vi "h.NET.GetNetworkIpMode.vi"(0 "Connection ID":refnum<k5>, 1 "error in":errorcluster) -> (2 "Connection ID":refnum<k5>, 3 "Network Mode":T1, 4 "Message":string, 5 "error out":errorcluster)   [LabVIEW 2016, in "h.Library.lvlib"]
doc: "This vi retrieves the current network settings.\n\n<b>Connection ID</b> - is a network connection refnum that uniquely identifies the TCP connection\n<b>error in</b> - describes error conditions that occur before this node runs. This input provides standard error functionality\n<b>Connection ID out</b> - returns the same value as connection ID\n<b>Network Mode</b> - returned network mode (either Static or DHCP)\n<b>Message</b> - human readable messages returned by the executed command\n<b>error out</b> - contains error information. This output provides standard error out functionality."
uses:
  h.Library.lvlib
  CTL/h.NET.NetworkMode.ctl
panel:
  # "Hyperion Get Network Configuration Mode"
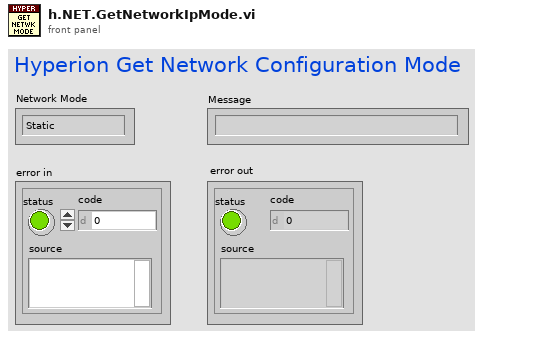
[diagram p1: front panel]
types:
  T1 = typedef "h.Library.lvlib/h.NET.NetworkMode.ctl" = enum8{"Static", "DHCP"}
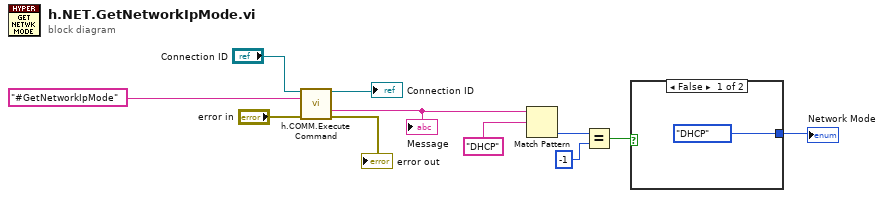
[diagram p0: block diagram]
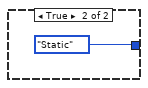
[diagram p2: hidden frame]
diagram:
  n1 = call "h.COMM.Execute Command.vi"("Connection ID"="Connection ID", "Command"="#GetNetworkIpMode", "error in"="error in") -> ("Connection ID out"=→"Connection ID":refnum<k5>, "Message"=w6:string, "error out"=→"error out":errorcluster)  [unwired: 5 in, 5 out]
  "Message" <- w6
  n2 = Match Pattern(string=w6, regular expression="DHCP" ("search string")) -> (offset past match=w4:i32)  [unwired: 1 in, 3 out]
  n3 = Equal?(x=w4, y=-1) -> (x = y?=w2:bool)
  n4 = case shown="False" w2 {
    tunnel: [h.NET.NetworkMode."DHCP" ("Network Mode") h.NET.NetworkMode."Static" ("Network Mode")] -> w1
    frame False {
    }
    frame True {
    }
  }
  "Network Mode" <- w1
